vi "Exercise_Traverse.vi"() -> ()   [LabVIEW 2010]
uses:
  Anemometry Sub Vis/Controls/Tunnel_Coordinates.ctl
  Anemometry Sub Vis/Controls/User_Specific_mode.ctl
  Anemometry Sub Vis/Gen Trav/Trav_mode.ctl
  Anemometry Sub Vis/Globals/Trav_pos_global.vi
panel:
  in  "Work in Tunnel Coordinates":T1
  in  "Number of travels":i32
  in  "End":dbl[](array[numeric])=[0.0, 0.0, 0.0] format="%#.2f"
  in  "Start":dbl[](array[numeric])=[0.0, 0.0, 0.0] format="%#.2f"
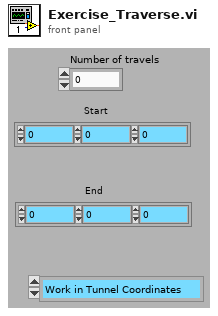
[diagram p1: front panel]
types:
  T1 = typedef "Tunnel_Coordinates.ctl" = enum16{"Work in Tunnel Coordinates", "Work in Model Coordinates"}
  T2 = typedef "User_Specific_mode.ctl" = enum16{"Check VI only", "Run VI"}
  T3 = typedef "Trav_mode.ctl" = enum16{"Move traverse", "Read traverse position", "Teach Position"}
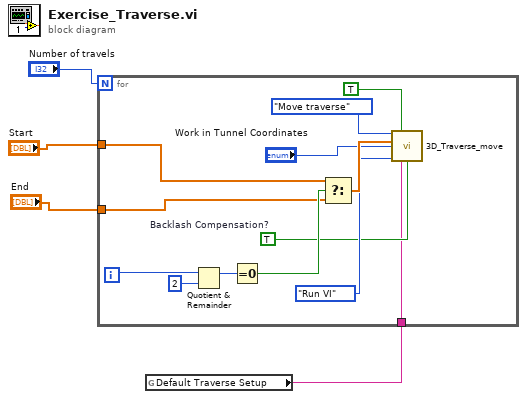
[diagram p0: block diagram]
diagram:
  n1 = global read "Trav_pos_global.vi" "Default Traverse Setup"() -> (w1:string)
  n2 = for {
    N: "Number of travels" -> [_]
    tunnel: "Start" -> [w12]
    tunnel: "End" -> [w11]
    tunnel: w1 -> [w5]
    i -> [w16]
    w6 = TRUE  # Backlash Compensation?
    n3 = Quotient & Remainder(x=w16, y=2) -> (x-y*floor(x/y)=w14:i32)  [unwired: 1 out]
    n4 = Equal To 0?(x=w14) -> (x = 0?=w13:bool)
    n5 = Select(t=w12, s=w13, f=w11) -> (s? t:f=w10:dbl[])
    n6 = call "3D_Traverse_move.vi"("Mode"=Trav_mode."Move traverse", "Route Checking?"=TRUE, "Position"=w10, "Work in Tunnel Coordinates"="Work in Tunnel Coordinates", "Simulate/Run"=User_Specific_mode."Run VI", "Traverse name"=w5, "Backlash Compensation?"=w6) -> ()  [unwired: 6 in, 3 out]
  }
